vi "Add to Array if Not Present (Variant).vi"(4 "Variant":variant, 5 "Variant Array":variant[](array[variant])) -> (1 "New Variant Array":variant[](array[variant]))   [LabVIEW 2011]
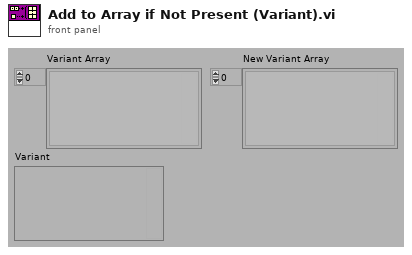
[diagram p1: front panel]
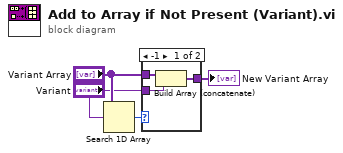
[diagram p0: block diagram]
diagram:
  n1 = Search 1D Array(1D array="Variant Array", element="Variant") -> (index of element=w4:i32)  [unwired: 1 out]
  n2 = case shown="-1" w4 {
    tunnel: "Variant Array" -> [w7 w8]
    tunnel: "Variant" -> [w6 _]
    tunnel: [w5 w8] -> w1
    frame -1 {
      n3 = Build Array (concatenate)(w7, w6) -> (w5:variant[])
    }
    frame Default {
    }
  }
  "New Variant Array" <- w1
